vi "Resize Subpanel Height.vi"(8 "error in (no error)":errorcluster, 9 "Height":u32, 10 "Subpanel Name":string, 11 "UI Controller in":refnum<class "UI Controller.lvclass">) -> (0 "error out":errorcluster, 3 "UI Controller out":refnum<class "UI Controller.lvclass">)   [LabVIEW 2020, in "UI Controller.lvlib" / "UI Controller.lvclass"]
uses:
  UI Controller.lvclass
  C:/Program Files/National Instruments/LabVIEW 2020/vi.lib/ActorFrameworkMVC/View Controller/View Controller/View Controller.lvclass
  <vilib>/ActorFrameworkMVC/View Controller/View Controller/View Controller.lvclass
panel:
  # "NOTICE -- YOU MUST LEAVE THIS NOTICE IN PLACE.\n\nCopyright (c) 2017, LIANG LIU Shawn.Liu.cn@gmail.com\nAll rights reserved.\n\nRedistribution and use in source and binary forms, with or without modification, are permitted provided that the following conditions are met:\n-Redistributions of source code must retain the above copyright notice, this list of conditions and the following disclaimer.\n-Redistributions in binary form must reproduce the above copyright notice, this list of conditions and the following disclaimer in the documentation and/or other materials provided with the distribution.\n-Neither the name of the eLp nor the names of its contributors may be used to endorse or promote products derived from this software without specific prior written permission.\n\nTHIS SOFTWARE IS PROVIDED BY THE COPYRIGHT HOLDERS AND CONTRIBUTORS \"AS IS\" AND ANY EXPRESS OR IMPLIED WARRANTIES, INCLUDING, BUT NOT LIMITED TO, THE IMPLIED WARRANTIES OF MERCHANTABILITY AND FITNESS FOR A PARTICULAR PURPOSE ARE DISCLAIMED. IN NO EVENT SHALL THE COPYRIGHT HOLDER OR CONTRIBUTORS BE LIABLE FOR ANY DIRECT, INDIRECT, INCIDENTAL, SPECIAL, EXEMPLARY, OR CONSEQUENTIAL DAMAGES (INCLUDING, BUT NOT LIMITED TO, PROCUREMENT OF SUBSTITUTE GOODS OR SERVICES; LOSS OF USE, DATA, OR PROFITS; OR BUSINESS INTERRUPTION) HOWEVER CAUSED AND ON ANY THEORY OF LIABILITY, WHETHER IN CONTRACT, STRICT LIABILITY, OR TORT (INCLUDING NEGLIGENCE OR OTHERWISE) ARISING IN ANY WAY OUT OF THE USE OF THIS SOFTWARE, EVEN IF ADVISED OF THE POSSIBILITY OF SUCH DAMAGE."
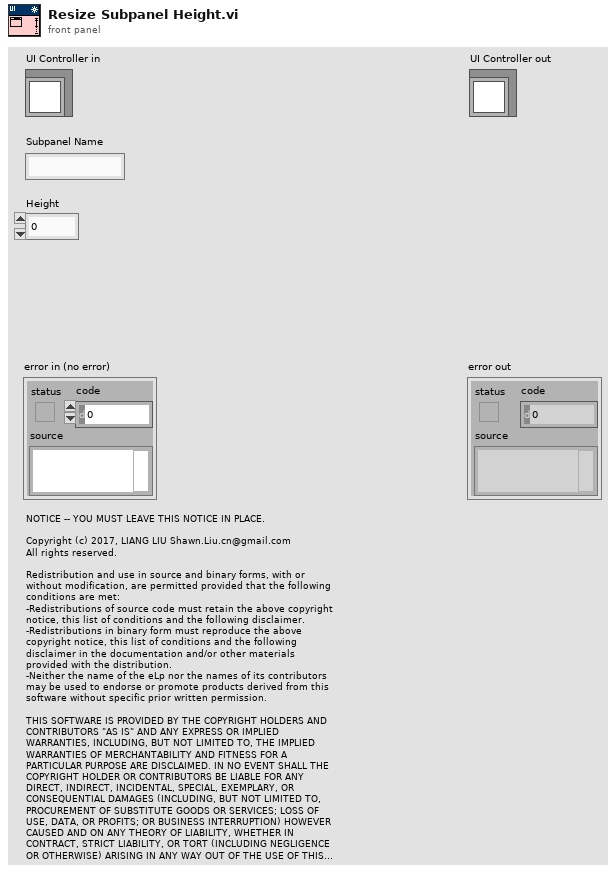
[diagram p1: front panel]
types:
  T1 = typedef "LVBoundsTypeDef.ctl" = cluster{"Width":u32, "Height":u32}
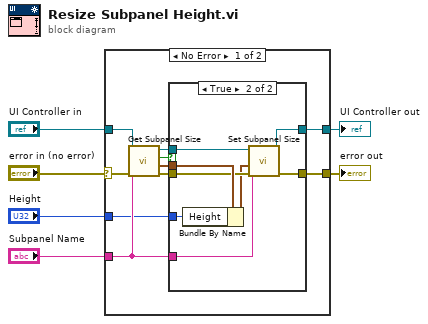
[diagram p0: block diagram]
diagram:
  n1 = case shown="No Error" "error in (no error)" {
    selector: "error in (no error)" -> [w9 w28]
    tunnel: [w16 w27] -> w6
    tunnel: "Subpanel Name" -> [w12 _]
    tunnel: "Height" -> [w11 _]
    tunnel: "UI Controller in" -> [w10 w27]
    tunnel: [w7 w28] -> w1
    frame No Error {
      n2 = call <vilib>:"Get Subpanel Size.vi"("error in (no error)"=w9, "Subpanel Name"=w12, "View Controller in"=w10) -> ("error out"=w8:errorcluster, "Subpanel Size"=w13:T1, "Found?"=w14:bool, "View Controller out"=w15:refnum<class "UI Controller.lvclass">)  [unwired: 5 in]
      n3 = case shown="True" w14 {
        tunnel: [w17 w22] -> w16
        tunnel: w15 -> [w17 w26]
        tunnel: w13 -> [_ w25]
        tunnel: w12 -> [_ w24]
        tunnel: w11 -> [_ w23]
        tunnel: w8 -> [w18 w21]
        tunnel: [w18 w20] -> w7
        frame False {
        }
        frame True {
          n4 = Bundle By Name(cluster=w25, "Height"=w23) -> (w19:T1)
          n5 = call <vilib>:"Set Subpanel Size.vi"("error in (no error)"=w21, "Subpanel Size"=w19, "Subpanel Name"=w24, "View Controller in"=w26) -> ("error out"=w20:errorcluster, "View Controller out"=w22:refnum<class "UI Controller.lvclass">)  [unwired: 5 in, 1 out]
        }
      }
    }
    frame Error {
    }
  }
  "error out" <- w1
  "UI Controller out" <- w6
